vi "Load Trigger Model Configuration Lists.vi"(0 "VISA resource name":refnum<visa-resource-name>, 1 "Measure Configuration List":string, 2 "Source Configuration List":string="MyMeasList", 3 "Enable Delay (F:False)":bool, 4 "Delay (0.000050)":dbl=5e-05 format="%#.6g", 5 "error in (no error)":errorcluster, 6 "Enable Buffer Name (F:False)":bool, 7 "Buffer Name (defbuffer1)":string="defbuffer1") -> (14 "VISA resource name out":refnum<visa-resource-name>, 19 "error out":errorcluster)   [LabVIEW 2020, in "Keithley 2450.lvlib"]
doc: "Loads a predefined trigger model configuration that uses source and measure configuration lists and optionally a delay and buffer name."
uses:
  <instrlib>/Keithley 2450/Keithley 2450.lvlib
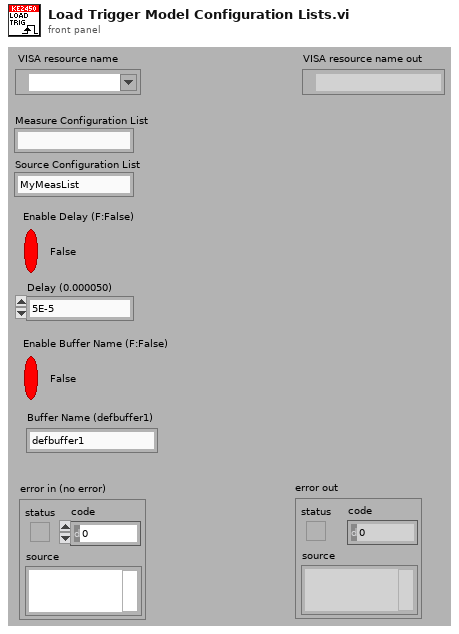
[diagram p1: front panel]
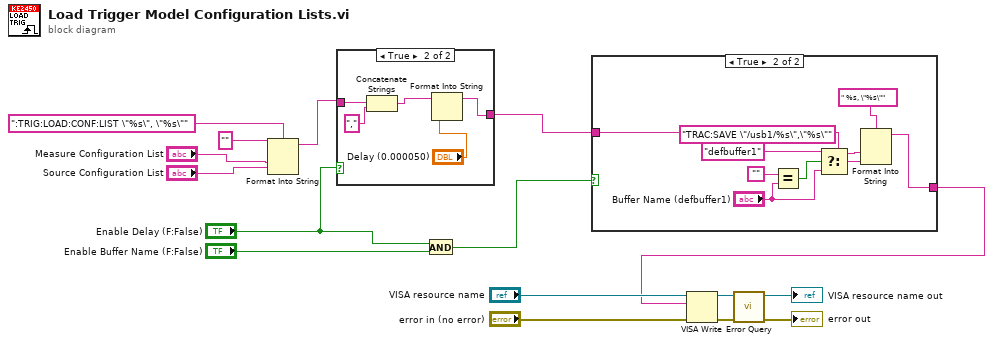
[diagram p0: block diagram]
diagram:
  (unwired) "TRAC:SAVE \"/usb1/%s\",\"%s\"" ("Read Measurement")
  n1 = Format Into String(format string=":TRIG:LOAD:CONF:LIST \"%s\", \"%s\"", initial string="", "Measure Configuration List", "Source Configuration List") -> (resulting string=w6:string)  [unwired: 1 in, 1 out]
  n2 = case shown="True" "Enable Delay (F:False)" {
    tunnel: [w17 w22] -> w1
    tunnel: w6 -> [w17 w20]
    frame False {
    }
    frame True {
      n3 = Concatenate Strings(w20, "," ("string")) -> (w18:string)
      n4 = Format Into String(initial string=w18, "Delay (0.000050)") -> (resulting string=w22:string)  [unwired: 2 in, 1 out]
    }
  }
  n5 = And(x="Enable Delay (F:False)", y="Enable Buffer Name (F:False)") -> (x .and. y?=w3:bool)
  n6 = case shown="True" w3 {
    tunnel: [w23 w26] -> w5
    tunnel: w1 -> [w23 w25]
    frame False {
    }
    frame True {
      n7 = Equal?(x="", y="Buffer Name (defbuffer1)") -> (x = y?=w29:bool)
      n8 = Select(t="defbuffer1", s=w29, f="Buffer Name (defbuffer1)") -> (s? t:f=w24:string)
      n9 = Format Into String(format string=" %s, \"%s\"" ("Read Measurement"), w25, w24) -> (resulting string=w26:string)  [unwired: 2 in, 1 out]
    }
  }
  n10 = VISA Write(VISA resource name="VISA resource name", write buffer=w5, error in (no error)="error in (no error)") -> (VISA resource name out=w12:refnum<visa-resource-name>, error out=w11:errorcluster)  [unwired: 1 out]
  n11 = call <instrlib>:"Error Query.vi"("error in (no error)"=w11, "VISA resource name"=w12) -> ("error out"=→"error out":errorcluster, "VISA resource name out"=→"VISA resource name out":refnum<visa-resource-name>)  [unwired: 8 out]
